vi "bson_finish.vi"(11 "cmd in":T1) -> (3 "cmd out":T1)   [LabVIEW 2013]
uses:
  bson.ctl
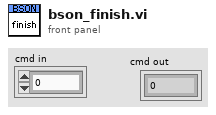
[diagram p1: front panel]
types:
  T1 = typedef "bson.ctl" = cluster{i32}
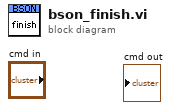
[diagram p0: block diagram]
diagram:
